vi "Configure Horizontal.vi"(8 "error in (no error)":errorcluster, 11 "object in":refnum<class "Fetch Display CFG.lvclass">) -> (0 "error out":errorcluster, 3 "object out":refnum<class "Fetch Display CFG.lvclass">)   [LabVIEW 2023, in "OWON SDS1022.lvlib" / "SDS1022 Base CFG.lvclass"]
uses:
  SDS1022 Base CFG.lvclass
  Fetch Display CFG/Fetch Display CFG.lvclass
  SDS1022 Base CFG.lvclass/SDS1022 Base CFG.ctl
  <instrlib>/OWON SDS1022/OWON SDS1022 Driver.lvlib
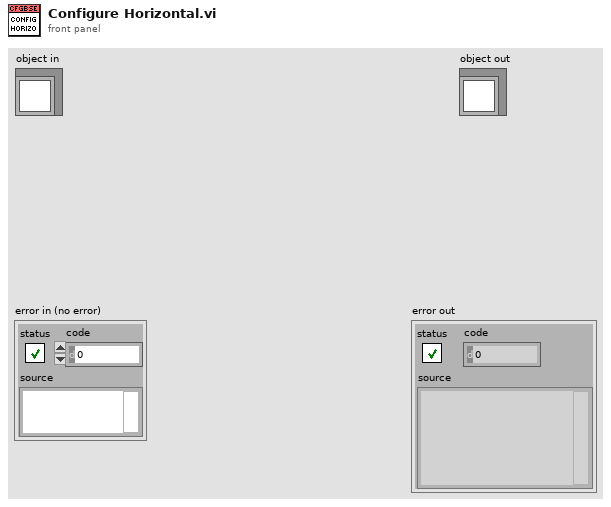
[diagram p1: front panel]
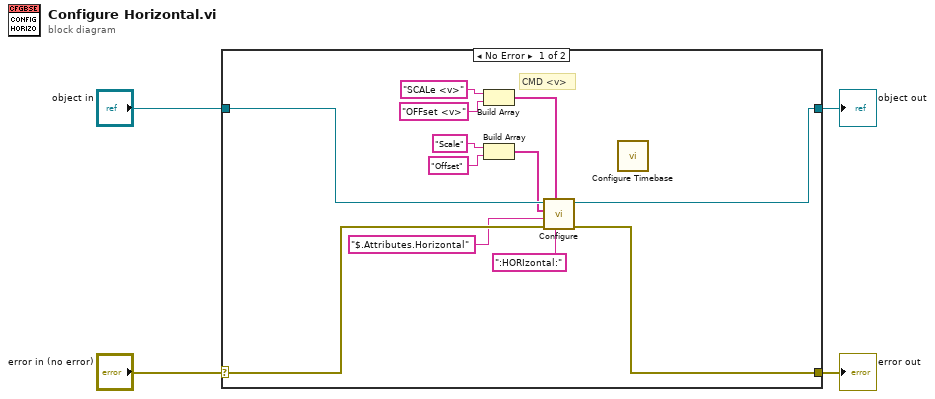
[diagram p0: block diagram]
diagram:
  n1 = case shown="No Error" "error in (no error)" {
    selector: "error in (no error)" -> [w16 w18]
    tunnel: [w15 w18] -> w3
    tunnel: [w5 w17] -> w1
    tunnel: "object in" -> [w10 w17]
    frame No Error {
      # "CMD <v>"
      n2 = Build Array("SCALe <v>" ("CMD Prefix"), "OFFset <v>" ("element")) -> (w12:string[])
      n3 = Build Array("Scale" ("CMD Prefix"), "Offset" ("element")) -> (w7:string[])
      n4 = call "Configure.vi"("CMD Prefix"=":HORIzontal:", "CMDs"=w12, "error in"=w16, "JSON Settings Path"="$.Attributes.Horizontal", "JSON Keys"=w7, "object in"=w10) -> ("error out"=w15:errorcluster, "object out"=w5:refnum<class "Fetch Display CFG.lvclass">)  [unwired: 4 in]
      n5 = call <instrlib>:"Configure Timebase.vi"() -> ()  [unwired: 10 in, 2 out]
    }
    frame Error {
    }
  }
  "error out" <- w3
  "object out" <- w1
